vi "SetRef.vi"(8 "error in (no error)":errorcluster, 10 "Set External":bool, 11 "PwrMtr_RSNRPZ in":refnum<class "PwrMtr_RSNRPZ.lvclass">) -> (0 "error out":errorcluster, 3 "PwrMtr_RSNRPZ out":refnum<class "PwrMtr_RSNRPZ.lvclass">)   [LabVIEW 2014, in "PwrMtr_RSNRPZ.lvclass"]
uses:
  PwrMtr_RSNRPZ.lvclass
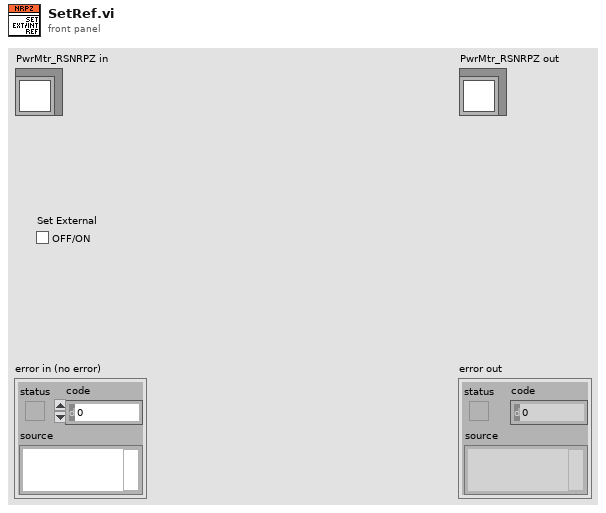
[diagram p1: front panel]
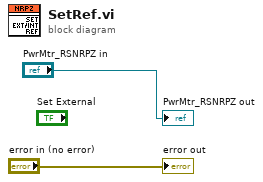
[diagram p0: block diagram]
diagram:
  "error out" <- "error in (no error)"
  "PwrMtr_RSNRPZ out" <- "PwrMtr_RSNRPZ in"
